vi "LakeShore 370 Write Setpoint.vi"(8 "error in (no error)":errorcluster, 10 "Output":dbl, 11 "VISA Refnum in":refnum<visa-resource-name>) -> (0 "error out":errorcluster)   [LabVIEW 2019]
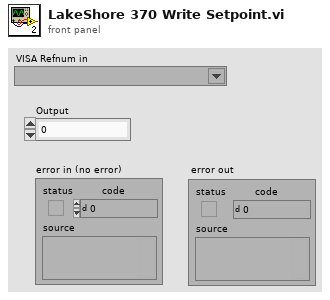
[diagram p1: front panel]
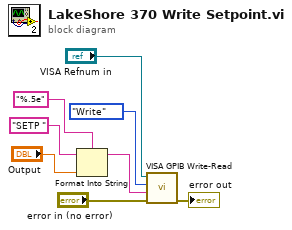
[diagram p0: block diagram]
diagram:
  n1 = Format Into String(format string="%.5e", initial string="SETP " ("format string"), "Output") -> (resulting string=w6:string)  [unwired: 1 in, 1 out]
  n2 = call "VISA GPIB Write-Read.vi"("error in (no error)"="error in (no error)", "Command"=w6, "Action"=enum16{"Write", "Read", "Write & Read"}."Write", "VISA resource name"="VISA Refnum in") -> ("error out"=→"error out":errorcluster)  [unwired: 4 in, 3 out]
